vi "LoadCell Program Labview.vi"() -> ()   [LabVIEW 2026]
uses:
  <vilib>/Instr/_visa.llb/VISA Configure Serial Port (Instr).vi
panel:
  in  "scaling factor":dbl=0.26 format="%#_13g"
  in  "offset voltage":dbl=2.6 format="%#_13g"
  in  "millisecond multiple":u32
  out "Weight(kgs)":dbl
  out "Voltage Recorded":dbl
  out "Volt Array":dbl[](array[numeric])
  in  "stop":bool
  out "Bytes at Serial Port (<30)":u32
  in  "VISA COM Port":refnum<visa-resource-name>
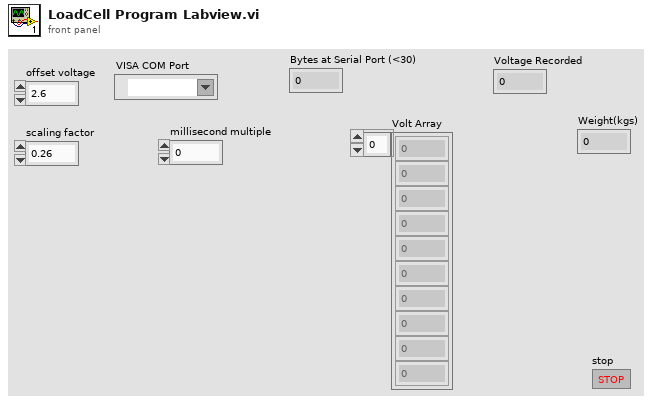
[diagram p1: front panel]
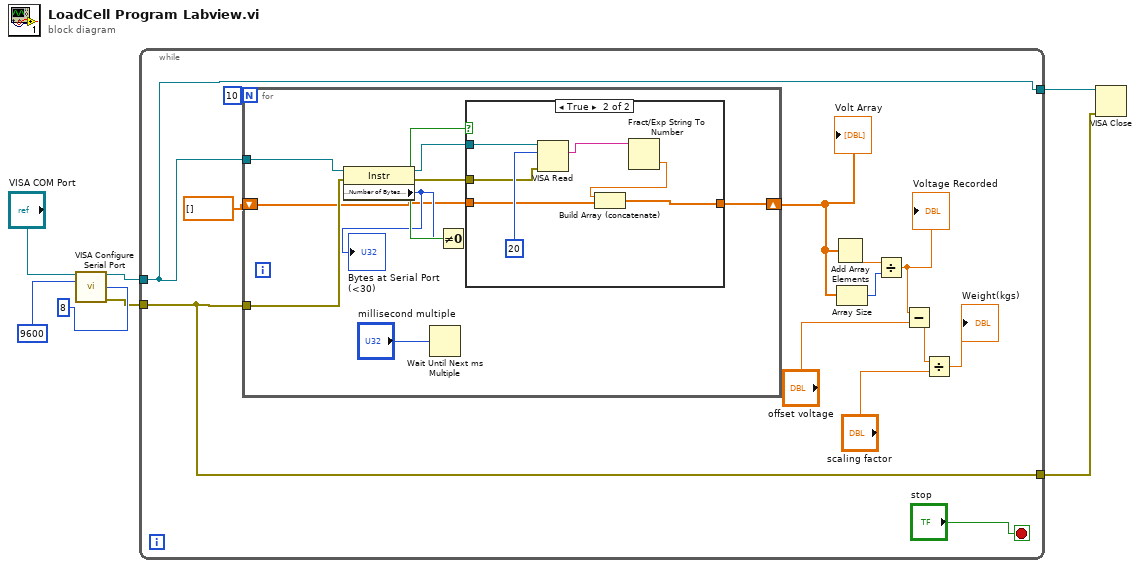
[diagram p0: block diagram]
diagram:
  n1 = call-poly "VISA Configure Serial Port"("VISA resource name"="VISA COM Port", "baud rate (9600)"=u32 9600, "data bits (8)"=u16 8) -> ("VISA resource name out"=w3:refnum<visa-resource-name>, "error out"=w4:errorcluster)  [unwired: 11 in]
  n2 = while {
    tunnel: w4 -> [w8]
    tunnel: w3 -> [w9]
    tunnel: [w9] -> w2
    tunnel: [w8] -> w1
    stop <- "stop" stop-if-true
    n3 = for {
      N: 10 ("Numeric") -> [_]
      tunnel: w9 -> [w29]
      tunnel: w8 -> [w28]
      shift-right: [w24] -> w15
      shift-left: dbl[] [] -> [w25]
      n4 = property class="Instr"(reference=w29, error in=w28) -> (reference out=w21:refnum<visa-resource-name>, error out=w22:errorcluster, "Serial Settings:Number of Bytes at Serial Port"=w26:u32)
      "Bytes at Serial Port (<30)" <- w26
      n5 = Wait Until Next ms Multiple(millisecond multiple="millisecond multiple") -> ()  [unwired: 1 out]
      n6 = Not Equal To 0?(x=w26) -> (x != 0?=w27:bool)
      n7 = case shown="True" w27 {
        tunnel: w25 -> [w30 w34]
        tunnel: [w30 w33] -> w24
        tunnel: w22 -> [_ w32]
        tunnel: w21 -> [_ w31]
        frame False {
        }
        frame True {
          n8 = VISA Read(VISA resource name=w31, byte count=u32 20, error in (no error)=w32) -> (read buffer=w36:string)  [unwired: 3 out]
          n9 = Fract/Exp String To Number(string=w36) -> (number=w35:dbl)  [unwired: 3 in, 1 out]
          n10 = Build Array (concatenate)(w35, w34) -> (w33:dbl[])
        }
      }
    }
    "Volt Array" <- w15
    n11 = Add Array Elements(numeric array=w15) -> (sum=w17:dbl)
    n12 = Array Size(array=w15) -> (size(s)=w16:i32)
    n13 = Divide(x=w17, y=w16) -> (x/y=w14:dbl)
    "Voltage Recorded" <- w14
    n14 = Subtract(x=w14, y="offset voltage") -> (x-y=w12:dbl)
    n15 = Divide(x=w12, y="scaling factor") -> (x/y=→"Weight(kgs)":dbl)
  }
  n16 = VISA Close(VISA resource name=w2, error in (no error)=w1) -> ()  [unwired: 1 out]
